vi "AD Detect Lv3 Overheat SPARKMAX.vi"(2 "Motors to test":string[](array[string]), 3 "Timing String":string) -> (0 "Disable Motors?":bool[](array[boolean]), 1 "Error Strings":string[](array[string]))   [LabVIEW 2019]
uses:
  <vilib>/ptbypt/NI_PtbyPt.lvlib
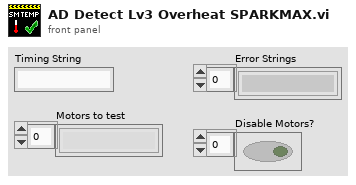
[diagram p1: front panel]
types:
  T1 = typedef "WPI_MotorControlDeviceRef.ctl" = cluster{"DeviceStatus":errorcluster, "Type":T2, "PWM":cluster{"PWM Channel":T3, "DeadBand":T4}, "CAN":cluster{"Device Number":u8, "SetOutput VI Ref":variant, "GetOutput VI Ref":variant, "Enable VI Ref":variant, "Disable VI Ref":variant, "Data":variant}, "Invert":bool, "DIO PWM":cluster{"PWM \"Enable\" Channel":T3, "DIOChannel":T5, "PWM Rate":dbl}}
  T2 = typedef "WPI_MotorControlType.ctl" = enum16{"PWM", "CAN", "DIO PWM"}
  T3 = typedef "FPGA_DIOPWMChannel.ctl" = enum8{"PWM 0", "PWM 1", "PWM 2", "PWM 3", "PWM 4", "PWM 5", "PWM 6", "PWM 7", "PWM 8", "PWM 9", "PWM MXP 0", "PWM MXP 1", "PWM MXP 2", "PWM MXP 3", "PWM MXP 4", "PWM MXP 5", "PWM MXP 6", "PWM MXP 7", "PWM MXP 8", "PWM MXP 9", "Invalid"}
  T4 = typedef "WPI_PWMDeadband.ctl" = cluster{"Name":string, "maxPositivePwm":i32, "minPositivePwm":i32, "centerPwm":i32, "maxNegativePwm":i32, "minNegativePwm":i32, "angularRange":u16}
  T5 = typedef "FPGA_DIOChannel.ctl" = enum8{"DIO 0", "DIO 1", "DIO 2", "DIO 3", "DIO 4", "DIO 5", "DIO 6", "DIO 7", "DIO 8", "DIO 9", "DIO MXP 0", "DIO MXP 1", "DIO MXP 2", "DIO MXP 3", "DIO MXP 4", "DIO MXP 5", "DIO MXP 6", "DIO MXP 7", "DIO MXP 8", "DIO MXP 9", "DIO MXP 10", "DIO MXP 11", "DIO MXP 12", "DIO MXP 13", "DIO MXP 14", "DIO MXP 15", "SPI Port CS1", "SPI Port CS2", "SPI Port CS3", "SPI Port MISO", "SPI Port MOSI", "Invalid"}
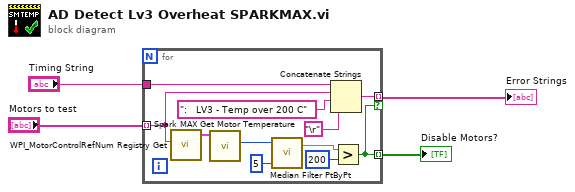
[diagram p0: block diagram]
diagram:
  n1 = for {
    tunnel: "Motors to test" -> [w9] mode=indexing
    tunnel: [w7] -> w2 mode=indexing if=w10
    tunnel: [w10] -> w1 mode=indexing
    tunnel: "Timing String" -> [w5]
    n2 = call <vilib>:"WPI_MotorControlRefNum Registry Get.vi"("refnum name"=w9) -> ("MotorControlDevRef"=w11:T1)  [unwired: 9 in, 1 out]
    n3 = call <vilib>:"Spark MAX Get Motor Temperature.vi"("MotorControlDevRef in"=w11) -> ("Motor Temperature"=w13:u8)  [unwired: 7 in, 3 out]
    n4 = call <vilib>:"Median Filter PtByPt.vi"("rank"=5, "x"=w13) -> ("Filtered x"=w12:dbl)  [unwired: 2 in, 1 out]
    n5 = Concatenate Strings(w5, w9, ":   LV3 - Temp over 200 C", "\r") -> (w7:string)
    n6 = Greater?(x=w12, y=u8 200) -> (0:w10:bool)
  }
  "Error Strings" <- w2
  "Disable Motors?" <- w1
